vi "Update Ball Pose.vi"(10 "x_k|k":T2, 11 "Detection Ball in":T1) -> (3 "Detection Ball out":T1)   [LabVIEW 2016]
uses:
  <vilib>/Analysis/Matrix/Datatypes/RealMatrix.ctl
  SSL Detection Ball.ctl
  <vilib>/Analysis/Matrix/NI_Matrix.lvlib
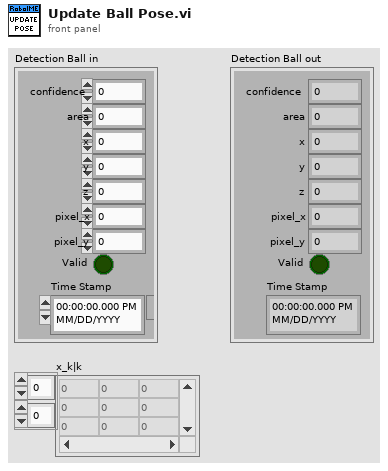
[diagram p1: front panel]
types:
  T1 = typedef "SSL Detection Ball.ctl" = cluster{"x":sgl, "area":u32, "confidence":sgl, "y":sgl, "z":sgl, "pixel_x":sgl, "pixel_y":sgl, "Valid":bool, "Time Stamp":timestamp}
  T2 = typedef "NI_Matrix.lvlib/RealMatrix.ctl" = dbl[][]
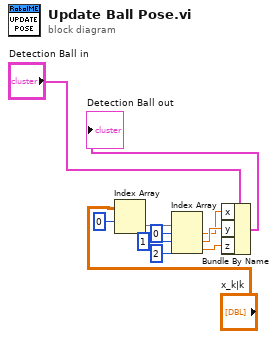
[diagram p0: block diagram]
diagram:
  n1 = Index Array(array="x_k|k", index (row)=0) -> (element=w4:dbl[])  [unwired: 1 in]
  n2 = Index Array(array=w4, index #1=0 ("index"), index #2=1 ("index"), index #3=2 ("index")) -> (element #1=w5:dbl, element #2=w6:dbl, element #3=w7:dbl)
  n3 = Bundle By Name(cluster="Detection Ball in", "x"=w5, "y"=w6, "z"=w7) -> (→"Detection Ball out":T1)
